vi "DOE Washer HCC Labels AGILENT.vi"(6 "Names":string[](array[string]), 8 "Error In":errorcluster, 9 "Agilent Data Input":dbl[](array[numeric])) -> (0 "Error Out":errorcluster, 3 "HCC Data Output":string[][](array[string]))   [LabVIEW 2016]
panel:
  in  "Station Name":string="HCC Row KNP"
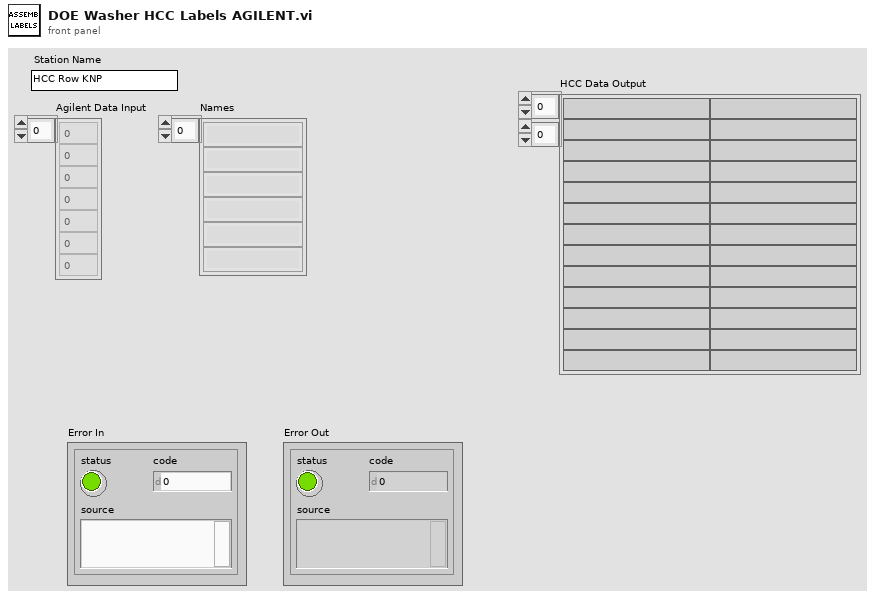
[diagram p1: front panel]
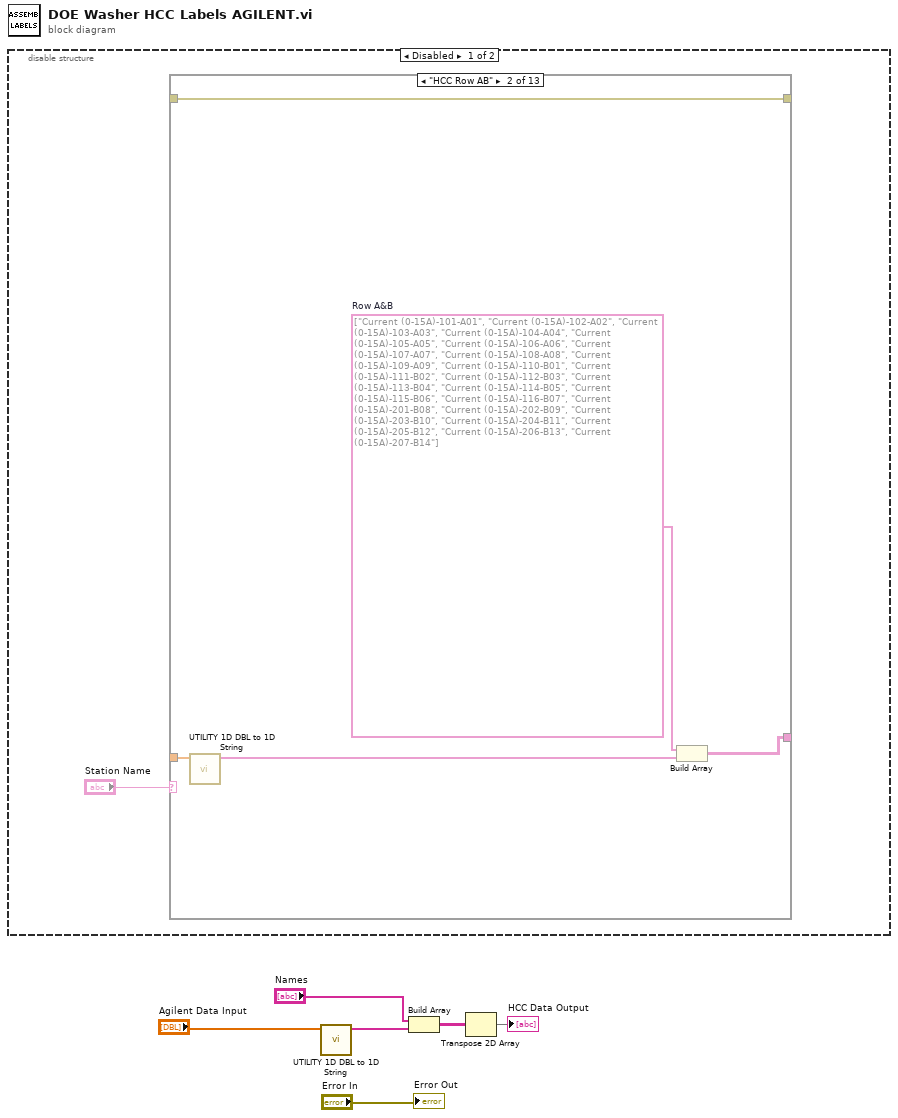
[diagram p0: block diagram]
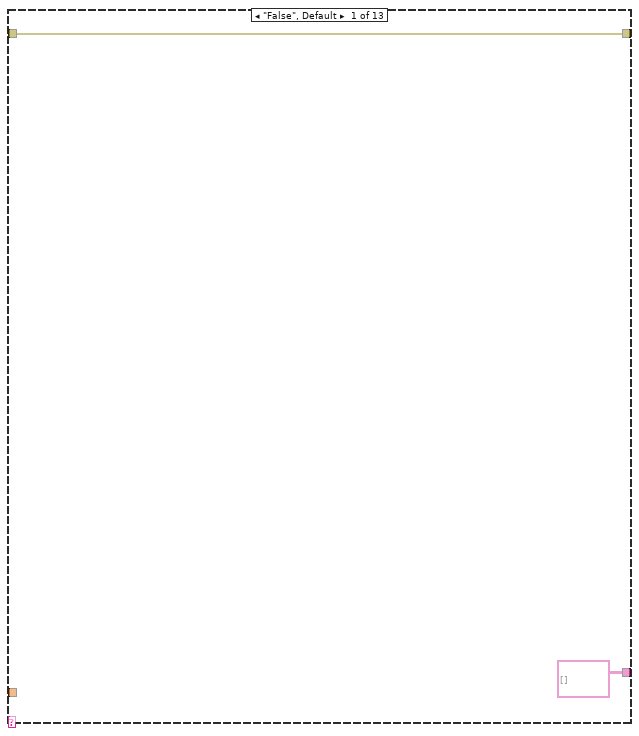
[diagram p2: hidden frame]
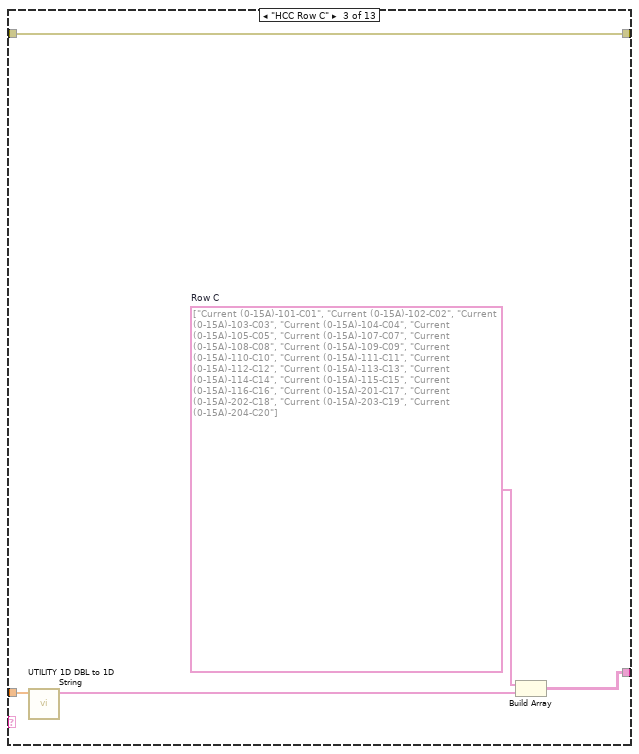
[diagram p3: hidden frame]
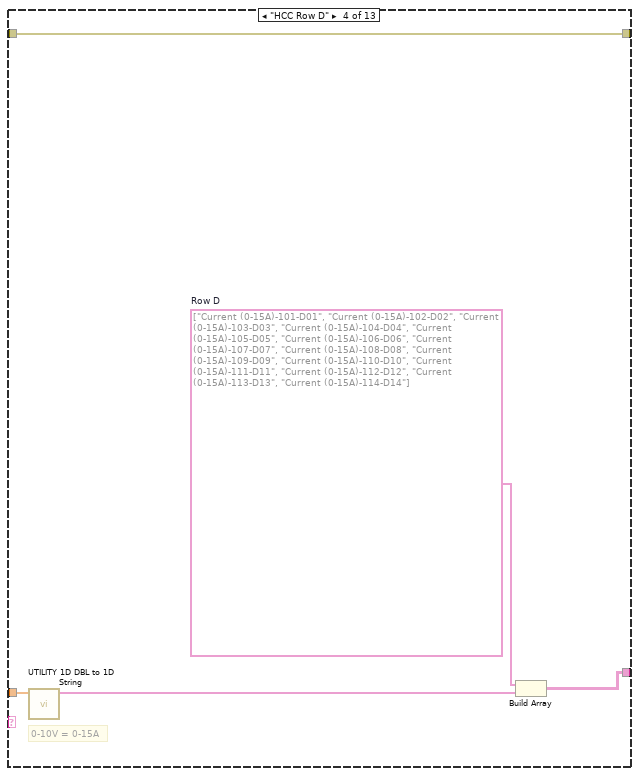
[diagram p4: hidden frame]
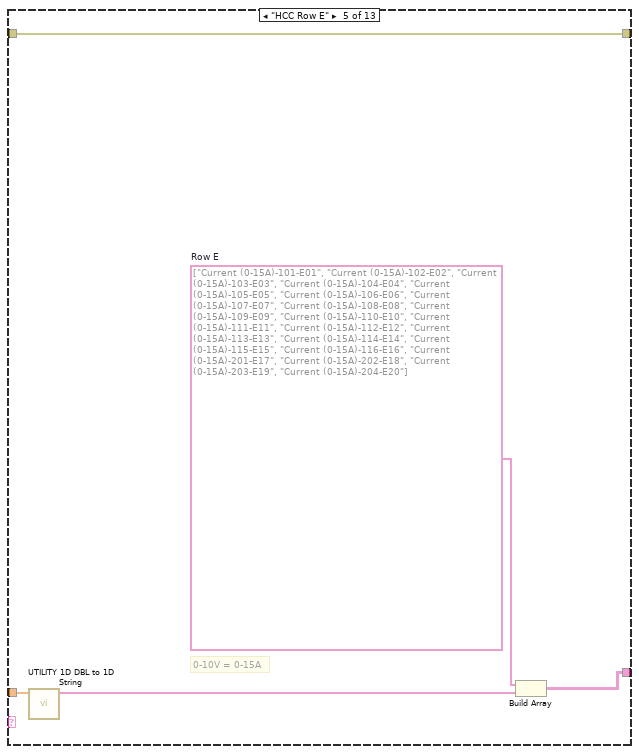
[diagram p5: hidden frame]
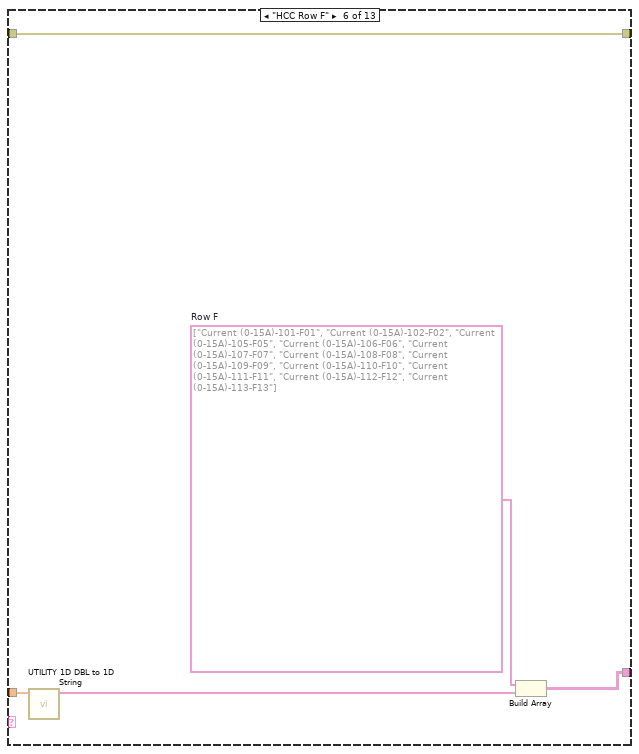
[diagram p6: hidden frame]
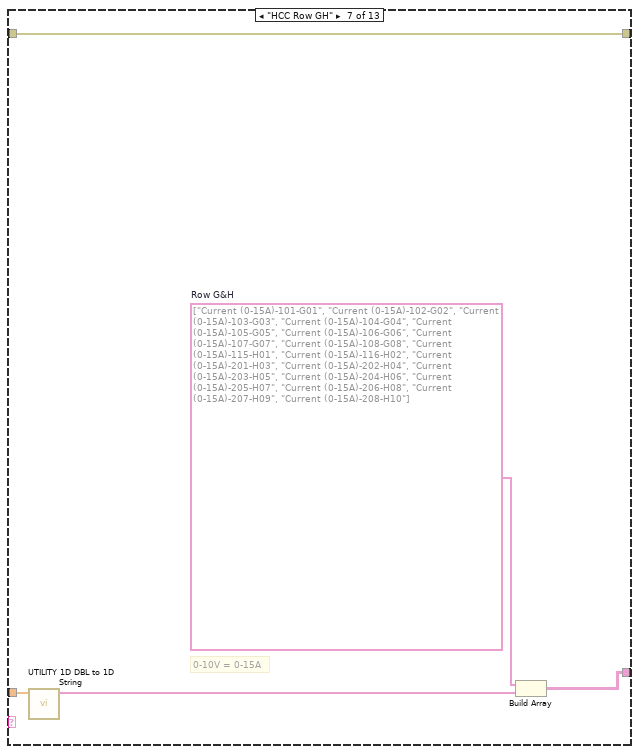
[diagram p7: hidden frame]
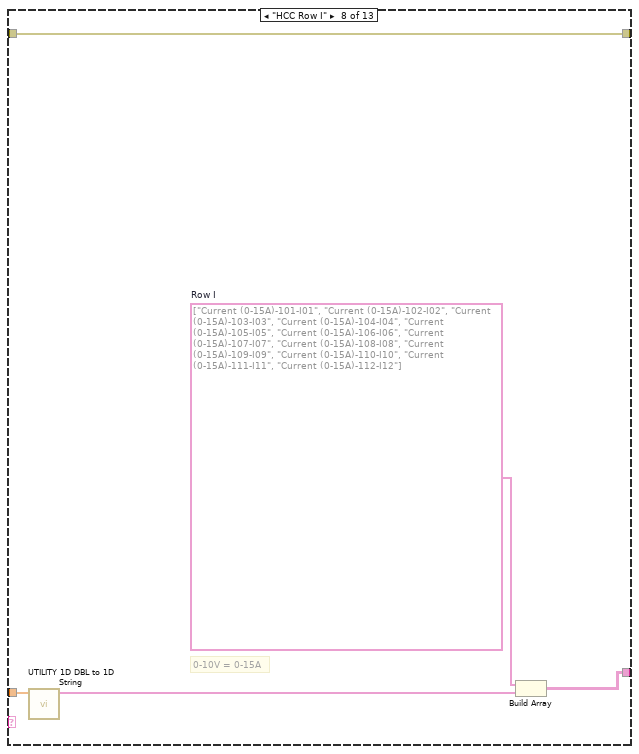
[diagram p8: hidden frame]
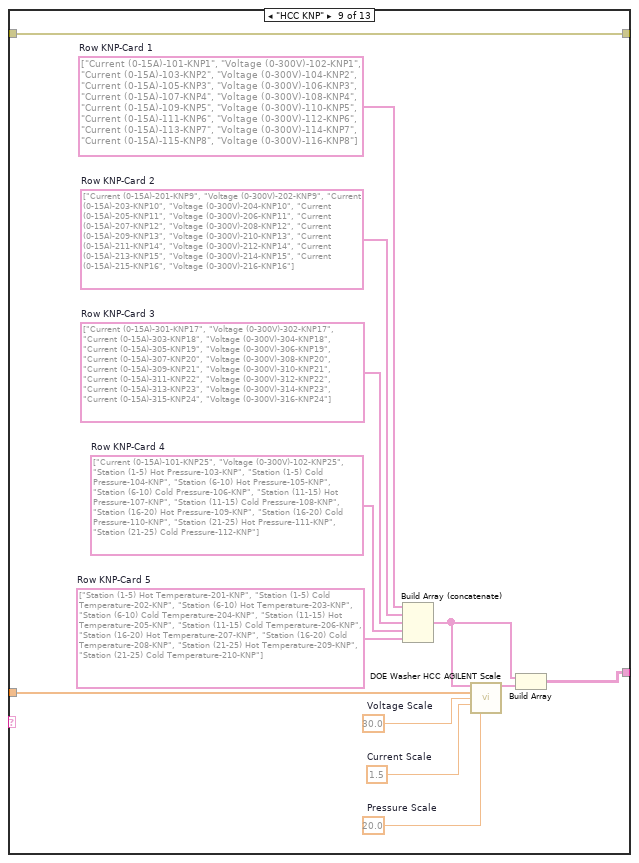
[diagram p9: hidden frame]
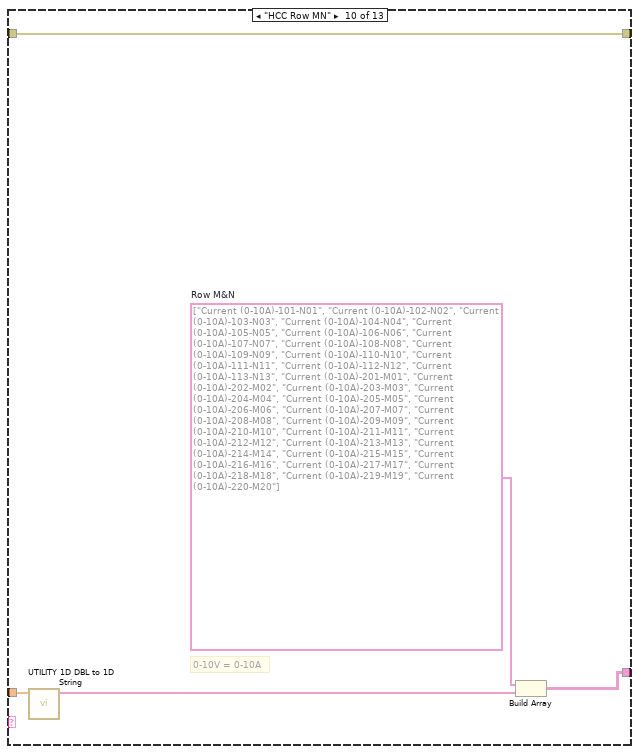
[diagram p10: hidden frame]
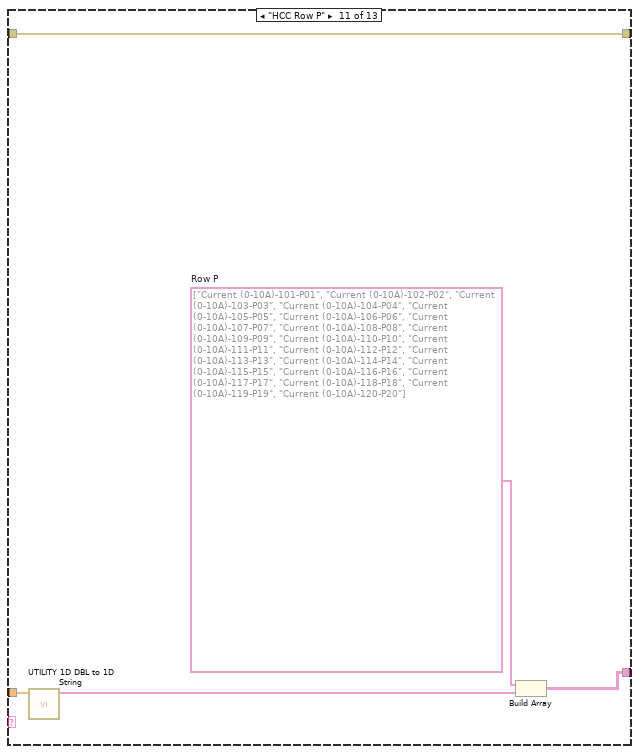
[diagram p11: hidden frame]
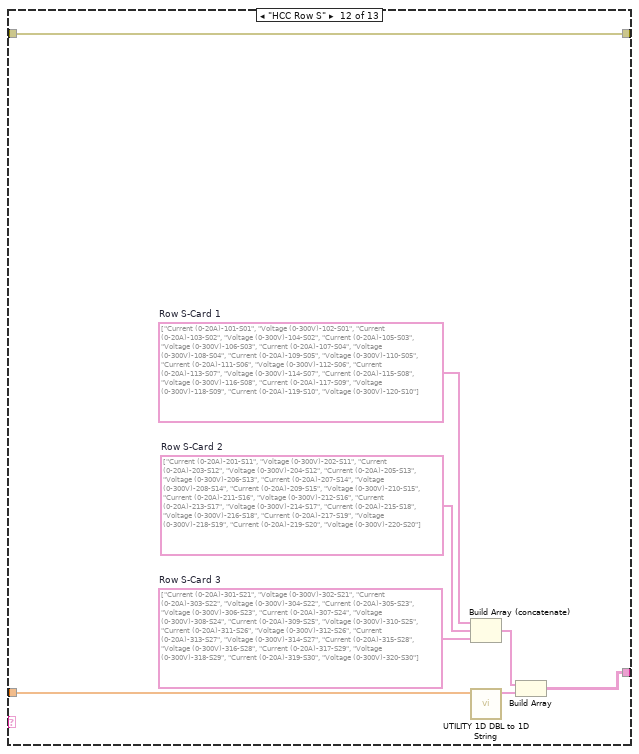
[diagram p12: hidden frame]
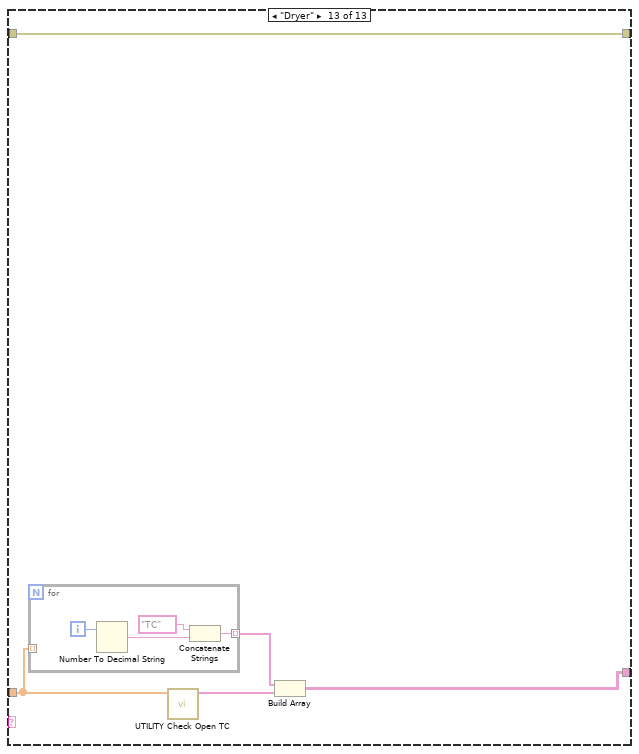
[diagram p13: hidden frame]
diagram:
  n1 = disable-structure shown="Disabled" {
    frame Disabled {
      n2 = case shown="\"HCC Row AB\"" "Station Name" {
        tunnel: _ -> [_ w10 w15 w20 w25 w30 w35 w40 w48 w58 w63 w68 w77]
        tunnel: [string[][] [] w12 w17 w21 w26 w31 w36 w41 w49 w60 w64 w70 w78] -> _
        tunnel: _ -> [w9 w11 w16 w24 w29 w34 w39 w44 w57 w59 w67 w75 w80]
        tunnel: [w9 w11 w16 w24 w29 w34 w39 w44 w57 w59 w67 w75 w80] -> _
        frame "False", Default {
        }
        frame "HCC Row AB" {
          w14 = string[] ["Current (0-15A)-101-A01", "Current (0-15A)-102-A02", "Current (0-15A)-103-A03", "Current (0-15A)-104-A04", "Current (0-15A)-105-A05", "Current (0-15A)-106-A06", "Current (0-15A)-107-A07", "Current (0-15A)-108-A08", "Current (0-15A)-109-A09", "Current (0-15A)-110-B01", "Current (0-15A)-111-B02", "Current (0-15A)-112-B03", "Current (0-15A)-113-B04", "Current (0-15A)-114-B05", "Current (0-15A)-115-B06", "Current (0-15A)-116-B07", "Current (0-15A)-201-B08", "Current (0-15A)-202-B09", "Current (0-15A)-203-B10", "Current (0-15A)-204-B11", "Current (0-15A)-205-B12", "Current (0-15A)-206-B13", "Current (0-15A)-207-B14"]  # Row A&B
          n3 = call "UTILITY 1D DBL to 1D String.vi"("1D DBL"=w10) -> ("1D String"=w13:string[])  [unwired: 10 in]
          n4 = Build Array(w14, w13) -> (w12:string[][])
        }
        frame "HCC Row C" {
          w19 = string[] ["Current (0-15A)-101-C01", "Current (0-15A)-102-C02", "Current (0-15A)-103-C03", "Current (0-15A)-104-C04", "Current (0-15A)-105-C05", "Current (0-15A)-107-C07", "Current (0-15A)-108-C08", "Current (0-15A)-109-C09", "Current (0-15A)-110-C10", "Current (0-15A)-111-C11", "Current (0-15A)-112-C12", "Current (0-15A)-113-C13", "Current (0-15A)-114-C14", "Current (0-15A)-115-C15", "Current (0-15A)-116-C16", "Current (0-15A)-201-C17", "Current (0-15A)-202-C18", "Current (0-15A)-203-C19", "Current (0-15A)-204-C20"]  # Row C
          n5 = call "UTILITY 1D DBL to 1D String.vi"("1D DBL"=w15) -> ("1D String"=w18:string[])  [unwired: 10 in]
          n6 = Build Array(w19, w18) -> (w17:string[][])
        }
        frame "HCC Row D" {
          w23 = string[] ["Current (0-15A)-101-D01", "Current (0-15A)-102-D02", "Current (0-15A)-103-D03", "Current (0-15A)-104-D04", "Current (0-15A)-105-D05", "Current (0-15A)-106-D06", "Current (0-15A)-107-D07", "Current (0-15A)-108-D08", "Current (0-15A)-109-D09", "Current (0-15A)-110-D10", "Current (0-15A)-111-D11", "Current (0-15A)-112-D12", "Current (0-15A)-113-D13", "Current (0-15A)-114-D14"]  # Row D
          # "0-10V = 0-15A"
          n7 = call "UTILITY 1D DBL to 1D String.vi"("1D DBL"=w20) -> ("1D String"=w22:string[])  [unwired: 10 in]
          n8 = Build Array(w23, w22) -> (w21:string[][])
        }
        frame "HCC Row E" {
          w28 = string[] ["Current (0-15A)-101-E01", "Current (0-15A)-102-E02", "Current (0-15A)-103-E03", "Current (0-15A)-104-E04", "Current (0-15A)-105-E05", "Current (0-15A)-106-E06", "Current (0-15A)-107-E07", "Current (0-15A)-108-E08", "Current (0-15A)-109-E09", "Current (0-15A)-110-E10", "Current (0-15A)-111-E11", "Current (0-15A)-112-E12", "Current (0-15A)-113-E13", "Current (0-15A)-114-E14", "Current (0-15A)-115-E15", "Current (0-15A)-116-E16", "Current (0-15A)-201-E17", "Current (0-15A)-202-E18", "Current (0-15A)-203-E19", "Current (0-15A)-204-E20"]  # Row E
          # "0-10V = 0-15A"
          n9 = call "UTILITY 1D DBL to 1D String.vi"("1D DBL"=w25) -> ("1D String"=w27:string[])  [unwired: 10 in]
          n10 = Build Array(w28, w27) -> (w26:string[][])
        }
        frame "HCC Row F" {
          w33 = string[] ["Current (0-15A)-101-F01", "Current (0-15A)-102-F02", "Current (0-15A)-105-F05", "Current (0-15A)-106-F06", "Current (0-15A)-107-F07", "Current (0-15A)-108-F08", "Current (0-15A)-109-F09", "Current (0-15A)-110-F10", "Current (0-15A)-111-F11", "Current (0-15A)-112-F12", "Current (0-15A)-113-F13"]  # Row F
          n11 = call "UTILITY 1D DBL to 1D String.vi"("1D DBL"=w30) -> ("1D String"=w32:string[])  [unwired: 10 in]
          n12 = Build Array(w33, w32) -> (w31:string[][])
        }
        frame "HCC Row GH" {
          w37 = string[] ["Current (0-15A)-101-G01", "Current (0-15A)-102-G02", "Current (0-15A)-103-G03", "Current (0-15A)-104-G04", "Current (0-15A)-105-G05", "Current (0-15A)-106-G06", "Current (0-15A)-107-G07", "Current (0-15A)-108-G08", "Current (0-15A)-115-H01", "Current (0-15A)-116-H02", "Current (0-15A)-201-H03", "Current (0-15A)-202-H04", "Current (0-15A)-203-H05", "Current (0-15A)-204-H06", "Current (0-15A)-205-H07", "Current (0-15A)-206-H08", "Current (0-15A)-207-H09", "Current (0-15A)-208-H10"]  # Row G&H
          # "0-10V = 0-15A"
          n13 = call "UTILITY 1D DBL to 1D String.vi"("1D DBL"=w35) -> ("1D String"=w38:string[])  [unwired: 10 in]
          n14 = Build Array(w37, w38) -> (w36:string[][])
        }
        frame "HCC Row I" {
          w43 = string[] ["Current (0-15A)-101-I01", "Current (0-15A)-102-I02", "Current (0-15A)-103-I03", "Current (0-15A)-104-I04", "Current (0-15A)-105-I05", "Current (0-15A)-106-I06", "Current (0-15A)-107-I07", "Current (0-15A)-108-I08", "Current (0-15A)-109-I09", "Current (0-15A)-110-I10", "Current (0-15A)-111-I11", "Current (0-15A)-112-I12"]  # Row I
          # "0-10V = 0-15A"
          n15 = call "UTILITY 1D DBL to 1D String.vi"("1D DBL"=w40) -> ("1D String"=w42:string[])  [unwired: 10 in]
          n16 = Build Array(w43, w42) -> (w41:string[][])
        }
        frame "HCC KNP" {
          w45 = string[] ["Station (1-5) Hot Temperature-201-KNP", "Station (1-5) Cold Temperature-202-KNP", "Station (6-10) Hot Temperature-203-KNP", "Station (6-10) Cold Temperature-204-KNP", "Station (11-15) Hot Temperature-205-KNP", "Station (11-15) Cold Temperature-206-KNP", "Station (16-20) Hot Temperature-207-KNP", "Station (16-20) Cold Temperature-208-KNP", "Station (21-25) Hot Temperature-209-KNP", "Station (21-25) Cold Temperature-210-KNP"]  # Row KNP-Card 5
          w46 = 20.0  # Pressure Scale
          w47 = string[] ["Current (0-15A)-101-KNP25", "Voltage (0-300V)-102-KNP25", "Station (1-5) Hot Pressure-103-KNP", "Station (1-5) Cold Pressure-104-KNP", "Station (6-10) Hot Pressure-105-KNP", "Station (6-10) Cold Pressure-106-KNP", "Station (11-15) Hot Pressure-107-KNP", "Station (11-15) Cold Pressure-108-KNP", "Station (16-20) Hot Pressure-109-KNP", "Station (16-20) Cold Pressure-110-KNP", "Station (21-25) Hot Pressure-111-KNP", "Station (21-25) Cold Pressure-112-KNP"]  # Row KNP-Card 4
          w52 = string[] ["Current (0-15A)-301-KNP17", "Voltage (0-300V)-302-KNP17", "Current (0-15A)-303-KNP18", "Voltage (0-300V)-304-KNP18", "Current (0-15A)-305-KNP19", "Voltage (0-300V)-306-KNP19", "Current (0-15A)-307-KNP20", "Voltage (0-300V)-308-KNP20", "Current (0-15A)-309-KNP21", "Voltage (0-300V)-310-KNP21", "Current (0-15A)-311-KNP22", "Voltage (0-300V)-312-KNP22", "Current (0-15A)-313-KNP23", "Voltage (0-300V)-314-KNP23", "Current (0-15A)-315-KNP24", "Voltage (0-300V)-316-KNP24"]  # Row KNP-Card 3
          w53 = string[] ["Current (0-15A)-201-KNP9", "Voltage (0-300V)-202-KNP9", "Current (0-15A)-203-KNP10", "Voltage (0-300V)-204-KNP10", "Current (0-15A)-205-KNP11", "Voltage (0-300V)-206-KNP11", "Current (0-15A)-207-KNP12", "Voltage (0-300V)-208-KNP12", "Current (0-15A)-209-KNP13", "Voltage (0-300V)-210-KNP13", "Current (0-15A)-211-KNP14", "Voltage (0-300V)-212-KNP14", "Current (0-15A)-213-KNP15", "Voltage (0-300V)-214-KNP15", "Current (0-15A)-215-KNP16", "Voltage (0-300V)-216-KNP16"]  # Row KNP-Card 2
          w54 = string[] ["Current (0-15A)-101-KNP1", "Voltage (0-300V)-102-KNP1", "Current (0-15A)-103-KNP2", "Voltage (0-300V)-104-KNP2", "Current (0-15A)-105-KNP3", "Voltage (0-300V)-106-KNP3", "Current (0-15A)-107-KNP4", "Voltage (0-300V)-108-KNP4", "Current (0-15A)-109-KNP5", "Voltage (0-300V)-110-KNP5", "Current (0-15A)-111-KNP6", "Voltage (0-300V)-112-KNP6", "Current (0-15A)-113-KNP7", "Voltage (0-300V)-114-KNP7", "Current (0-15A)-115-KNP8", "Voltage (0-300V)-116-KNP8"]  # Row KNP-Card 1
          w55 = 1.5  # Current Scale
          w56 = 30.0  # Voltage Scale
          n17 = Build Array (concatenate)(w54, w53, w52, w47, w45) -> (w51:string[])
          n18 = call "DOE Washer HCC AGILENT Scale.vi"("Headers"=w51, "Agilent Data Input"=w48, "Voltage Scale"=w56, "Current Scale"=w55, "Pressure Scale"=w46) -> ("Scaled Output Data"=w50:string[])  [unwired: 9 in, 1 out]
          n19 = Build Array(w51, w50) -> (w49:string[][])
        }
        frame "HCC Row MN" {
          w62 = string[] ["Current (0-10A)-101-N01", "Current (0-10A)-102-N02", "Current (0-10A)-103-N03", "Current (0-10A)-104-N04", "Current (0-10A)-105-N05", "Current (0-10A)-106-N06", "Current (0-10A)-107-N07", "Current (0-10A)-108-N08", "Current (0-10A)-109-N09", "Current (0-10A)-110-N10", "Current (0-10A)-111-N11", "Current (0-10A)-112-N12", "Current (0-10A)-113-N13", "Current (0-10A)-201-M01", "Current (0-10A)-202-M02", "Current (0-10A)-203-M03", "Current (0-10A)-204-M04", "Current (0-10A)-205-M05", "Current (0-10A)-206-M06", "Current (0-10A)-207-M07", "Current (0-10A)-208-M08", "Current (0-10A)-209-M09", "Current (0-10A)-210-M10", "Current (0-10A)-211-M11", "Current (0-10A)-212-M12", "Current (0-10A)-213-M13", "Current (0-10A)-214-M14", "Current (0-10A)-215-M15", "Current (0-10A)-216-M16", "Current (0-10A)-217-M17", "Current (0-10A)-218-M18", "Current (0-10A)-219-M19", "Current (0-10A)-220-M20"]  # Row M&N
          # "0-10V = 0-10A"
          n20 = call "UTILITY 1D DBL to 1D String.vi"("1D DBL"=w58) -> ("1D String"=w61:string[])  [unwired: 10 in]
          n21 = Build Array(w62, w61) -> (w60:string[][])
        }
        frame "HCC Row P" {
          w66 = string[] ["Current (0-10A)-101-P01", "Current (0-10A)-102-P02", "Current (0-10A)-103-P03", "Current (0-10A)-104-P04", "Current (0-10A)-105-P05", "Current (0-10A)-106-P06", "Current (0-10A)-107-P07", "Current (0-10A)-108-P08", "Current (0-10A)-109-P09", "Current (0-10A)-110-P10", "Current (0-10A)-111-P11", "Current (0-10A)-112-P12", "Current (0-10A)-113-P13", "Current (0-10A)-114-P14", "Current (0-10A)-115-P15", "Current (0-10A)-116-P16", "Current (0-10A)-117-P17", "Current (0-10A)-118-P18", "Current (0-10A)-119-P19", "Current (0-10A)-120-P20"]  # Row P
          n22 = call "UTILITY 1D DBL to 1D String.vi"("1D DBL"=w63) -> ("1D String"=w65:string[])  [unwired: 10 in]
          n23 = Build Array(w66, w65) -> (w64:string[][])
        }
        frame "HCC Row S" {
          w72 = string[] ["Current (0-20A)-301-S21", "Voltage (0-300V)-302-S21", "Current (0-20A)-303-S22", "Voltage (0-300V)-304-S22", "Current (0-20A)-305-S23", "Voltage (0-300V)-306-S23", "Current (0-20A)-307-S24", "Voltage (0-300V)-308-S24", "Current (0-20A)-309-S25", "Voltage (0-300V)-310-S25", "Current (0-20A)-311-S26", "Voltage (0-300V)-312-S26", "Current (0-20A)-313-S27", "Voltage (0-300V)-314-S27", "Current (0-20A)-315-S28", "Voltage (0-300V)-316-S28", "Current (0-20A)-317-S29", "Voltage (0-300V)-318-S29", "Current (0-20A)-319-S30", "Voltage (0-300V)-320-S30"]  # Row S-Card 3
          w73 = string[] ["Current (0-20A)-201-S11", "Voltage (0-300V)-202-S11", "Current (0-20A)-203-S12", "Voltage (0-300V)-204-S12", "Current (0-20A)-205-S13", "Voltage (0-300V)-206-S13", "Current (0-20A)-207-S14", "Voltage (0-300V)-208-S14", "Current (0-20A)-209-S15", "Voltage (0-300V)-210-S15", "Current (0-20A)-211-S16", "Voltage (0-300V)-212-S16", "Current (0-20A)-213-S17", "Voltage (0-300V)-214-S17", "Current (0-20A)-215-S18", "Voltage (0-300V)-216-S18", "Current (0-20A)-217-S19", "Voltage (0-300V)-218-S19", "Current (0-20A)-219-S20", "Voltage (0-300V)-220-S20"]  # Row S-Card 2
          w74 = string[] ["Current (0-20A)-101-S01", "Voltage (0-300V)-102-S01", "Current (0-20A)-103-S02", "Voltage (0-300V)-104-S02", "Current (0-20A)-105-S03", "Voltage (0-300V)-106-S03", "Current (0-20A)-107-S04", "Voltage (0-300V)-108-S04", "Current (0-20A)-109-S05", "Voltage (0-300V)-110-S05", "Current (0-20A)-111-S06", "Voltage (0-300V)-112-S06", "Current (0-20A)-113-S07", "Voltage (0-300V)-114-S07", "Current (0-20A)-115-S08", "Voltage (0-300V)-116-S08", "Current (0-20A)-117-S09", "Voltage (0-300V)-118-S09", "Current (0-20A)-119-S10", "Voltage (0-300V)-120-S10"]  # Row S-Card 1
          n24 = Build Array (concatenate)(w74, w73, w72) -> (w71:string[])
          n25 = call "UTILITY 1D DBL to 1D String.vi"("1D DBL"=w68) -> ("1D String"=w69:string[])  [unwired: 10 in]
          n26 = Build Array(w71, w69) -> (w70:string[][])
        }
        frame "Dryer" {
          n27 = for {
            tunnel: w77 -> [_] mode=indexing
            tunnel: [w81] -> w79 mode=indexing
            i -> [w83]
            n28 = Number To Decimal String(number=w83) -> (decimal integer string=w82:string)  [unwired: 1 in]
            n29 = Concatenate Strings("TC", w82) -> (w81:string)
          }
          n30 = call "UTILITY Check Open TC.vi"("Input TC Values"=w77) -> ("Updated TC Array"=w76:string[])  [unwired: 9 in, 1 out]
          n31 = Build Array(w79, w76) -> (w78:string[][])
        }
      }
    }
    frame Enabled {
    }
  }
  n32 = call "UTILITY 1D DBL to 1D String.vi"("1D DBL"="Agilent Data Input") -> ("1D String"=w4:string[])  [unwired: 10 in]
  n33 = Build Array("Names", w4) -> (w2:string[][])
  n34 = Transpose 2D Array(2D array=w2) -> (transposed array=→"HCC Data Output":string[][])
  "Error Out" <- "Error In"
